vi "ReadLogFile.vi"(10 "file name":string) -> (2 "Array":i32[](array[numeric]))   [LabVIEW 2018]
uses:
  <vilib>/Analysis/NI_AALBase.lvlib
panel:
  out "Histogram Graph":T1(graph)
  out "variance":dbl format="%0.2f"
  out "std dev":dbl format="%0.2f"
  out "mean":dbl format="%0.2f"
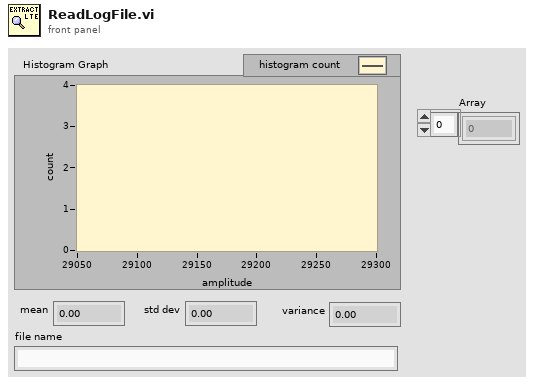
[diagram p1: front panel]
types:
  T1 = cluster{"X Values":dbl[], "Histogram: h(x)":i32[]}
  T2 = enum16{"open", "replace", "create", "open or create", "replace or create", "replace or create with confirmation"}
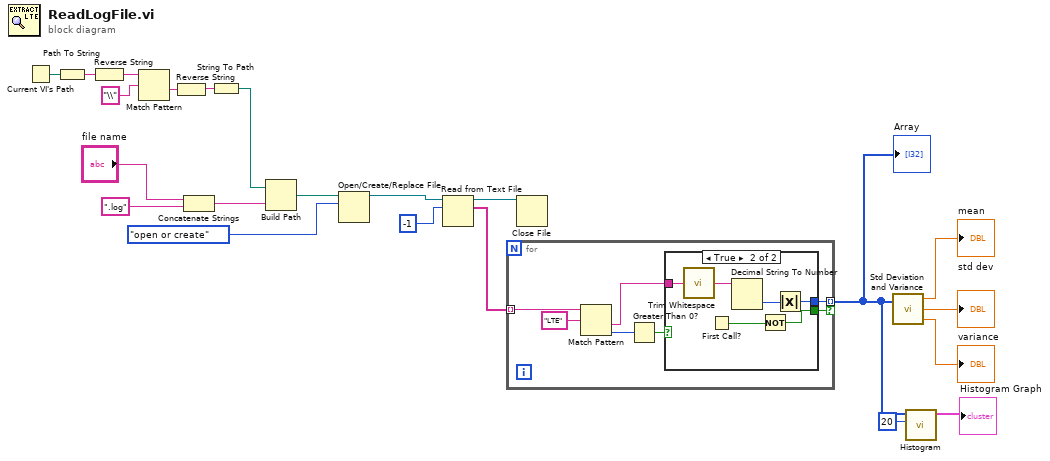
[diagram p0: block diagram]
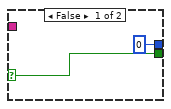
[diagram p2: hidden frame]
diagram:
  n1 = Current VI's Path() -> (path=w10:path)
  n2 = Path To String(path=w10) -> (string=w9:string)
  n3 = Reverse String(1:w9) -> (0:w8:string)
  n4 = Match Pattern(string=w8, regular expression="\\") -> (after substring=w12:string)  [unwired: 1 in, 3 out]
  n5 = Reverse String(1:w12) -> (0:w11:string)
  n6 = Concatenate Strings("file name", ".log" ("regular expression")) -> (w7:string)
  n7 = String To Path(string=w11) -> (path=w4:path)
  n8 = Build Path(base path=w4, name or relative path=w7) -> (appended path=w5:path)
  n9 = Open/Create/Replace File(file path (use dialog)=w5, operation (0:open)=T2."open or create") -> (refnum out=w2:refnum<file>)  [unwired: 4 in, 2 out]
  n10 = Read from Text File(file (use dialog)=w2, count=-1) -> (refnum out=w22:refnum<file>, text=w20:string[])  [unwired: 2 in, 2 out]
  n11 = for {
    tunnel: w20 -> [w29] mode=indexing
    tunnel: [w25] -> w16 mode=indexing if=w23
    n12 = Match Pattern(string=w29, regular expression="LTE") -> (after substring=w26:string, offset past match=w27:i32)  [unwired: 1 in, 2 out]
    n13 = Greater Than 0?(x=w27) -> (x > 0?=w24:bool)
    n14 = case shown="True" w24 {
      selector: w24 -> [w31 _]
      tunnel: w26 -> [_ w37]
      tunnel: [0 w35] -> w25
      tunnel: [w31 w32] -> w23
      frame False {
      }
      frame True {
        n15 = call <vilib>:"Trim Whitespace.vi"("string"=w37) -> ("trimmed string"=w34:string)  [unwired: 1 in]
        n16 = First Call?() -> (First Call?: T/F=w33:bool)
        n17 = Decimal String To Number(string=w34) -> (number=w36:i32)  [unwired: 2 in, 1 out]
        n18 = Not(x=w33) -> (.not. x?=w32:bool)
        n19 = Absolute Value(x=w36) -> (abs(x)=w35:i32)
      }
    }
  }
  "Array" <- w16
  n20 = Close File(refnum=w22) -> ()  [unwired: 1 in, 2 out]
  n21 = call <vilib>:"Std Deviation and Variance.vi"("X"=w16) -> ("mean"=→"mean":dbl, "standard deviation"=→"std dev":dbl, "variance"=→"variance":dbl)  [unwired: 1 in]
  n22 = call <vilib>:"Histogram.vi"("intervals"=20, "X"=w16) -> ("Histogram Graph"=→"Histogram Graph":T1)  [unwired: 6 in, 3 out]
